vi "NI VeriStand FPGA DMA IO.vi"() -> ()   [LabVIEW 2019]
uses:
  <vilib>/Platform/TimedLoop/XDataNode/wakeup.ctl
  <vilib>/Platform/TimedLoop/XDataNode/XDNodeRunTimeDep.lvlib
  <vilib>/Platform/TimedLoop/XDataNode/nitl_modes.ctl
  <vilib>/Platform/TimedLoop/XDataNode/timing_clust.ctl
  <vilib>/Platform/TimedLoop/XDataNode/XDataNode.xnode
  <vilib>/eio/EIONode/EIONode.xnode
  <vilib>/NI VeriStand/FPGA/NI_VS FPGA Support.lvlib
  <vilib>/eio/EIOMethodNode/EIOMethodNode.xnode
  <vilib>/rvi/eio/common/nirviEmuTemplateMethod_errors.vi
panel:
  in  "Generate IRQ":bool
  in  "Clock Pulse":bool
  in  "Clock Ticked":bool
  in  "Use External Timing":bool
  in  "Write to  RTSI":bool
  in  "Loop Rate (usec)":u32
  in  "Start":bool
  in  "_Low Pulse 7":u32
  in  "_High Pulse 7":u32
  in  "_Low Pulse 5":u32
  in  "_High Pulse 5":u32
  in  "_Low Pulse 6":u32
  in  "_High Pulse 6":u32
  in  "_Low Pulse 4":u32
  in  "_High Pulse 4":u32
  in  "_PWM In 7 timeout":u32=40000
  out "_PWM In 7 High Time":u32
  out "_PWM In 7 Low Time":u32
  in  "_PWM In 6 timeout":u32=40000
  out "_PWM In 6 High Time":u32
  out "_PWM In 6 Low Time":u32
  in  "_PWM In 5 timeout":u32=40000
  out "_PWM In 5 High Time":u32
  out "_PWM In 5 Low Time":u32
  in  "_PWM In 4 timeout":u32=40000
  out "_PWM In 4 High Time":u32
  out "_PWM In 4 Low Time":u32
  in  "_PWM In 3 timeout":u32=40000
  out "_PWM In 3 High Time":u32
  out "_PWM In 3 Low Time":u32
  in  "_PWM In 2 timeout":u32=40000
  out "_PWM In 2 High Time":u32
  out "_PWM In 2 Low Time":u32
  in  "_PWM In 1 timeout":u32=40000
  out "_PWM In 1 High Time":u32
  out "_PWM In 1 Low Time":u32
  in  "_PWM In 0 timeout":u32=40000
  out "_PWM In 0 High Time":u32
  out "_PWM In 0 Low Time":u32
  in  "_Low Pulse 3":u32
  in  "_High Pulse 3":u32
  in  "_Low Pulse 1":u32
  in  "_High Pulse 1":u32
  in  "_Low Pulse 2":u32
  in  "_High Pulse 2":u32
  in  "_Low Pulse 0":u32
  in  "_High Pulse 0":u32
  # "PWM"
  # "Configuration"
  # "Internal Controls"
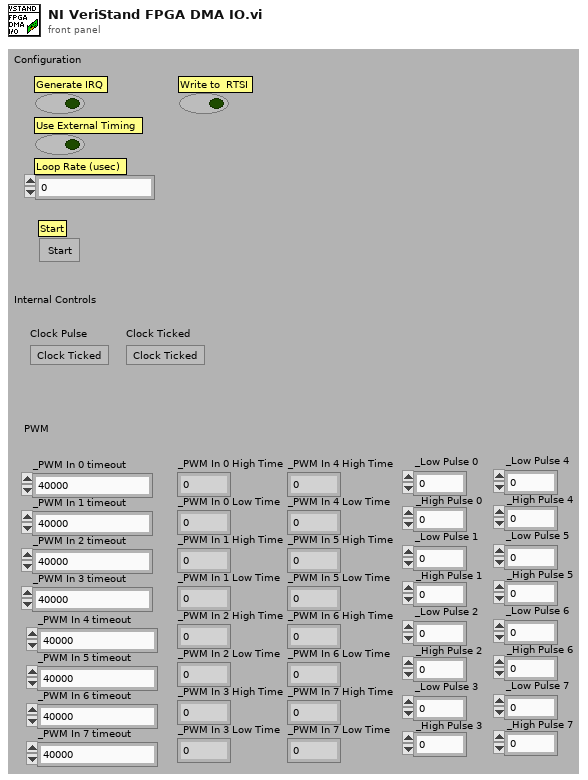
[diagram p1: front panel]
types:
  T1 = typedef "XDNodeRunTimeDep.lvlib/timing_clust.ctl" = cluster{"Expected End [f-1]":u64, "Actual End [f-1]":u64, "Finished Late? [f-1]":bool, "Expected End [i-1]":u64, "Actual End [i-1]":u64, "Finished Late? [i-1]":bool, "Expected Start [i]":u64, "Actual Start [i]":u64, "Expected Start [f]":u64, "Actual Start [f]":u64, "Source Name":string, "Structure Name":string, "Period":i64, "Deadline":i64, "Offset":i64, "Start":i64, "Priority":i32, "Timeout":i32, "Mode":T2, "Wakeup Reason":T3, "Error":errorcluster, "Source Type":string, "Secondary Source Type":string, "Global End Time":u64, "Global Start Time":u64, "Frame Duration":u64, "Iteration Duration":u64, "Assigned CPU":i32, "I/O Scan Engine Mode":u32}
  T2 = typedef "XDNodeRunTimeDep.lvlib/nitl_modes.ctl" = enum32{"No Change", "Process missed periods, maintain original phase", "Discard missed periods, maintain original phase", "Process missed periods, ignore original phase", "Discard missed periods, ignore original phase"}
  T3 = typedef "XDNodeRunTimeDep.lvlib/wakeup.ctl" = enum32{"Normal", "Aborted", "Asynchronous wakeup", "Timing source error", "Timed loop error", "Timeout"}
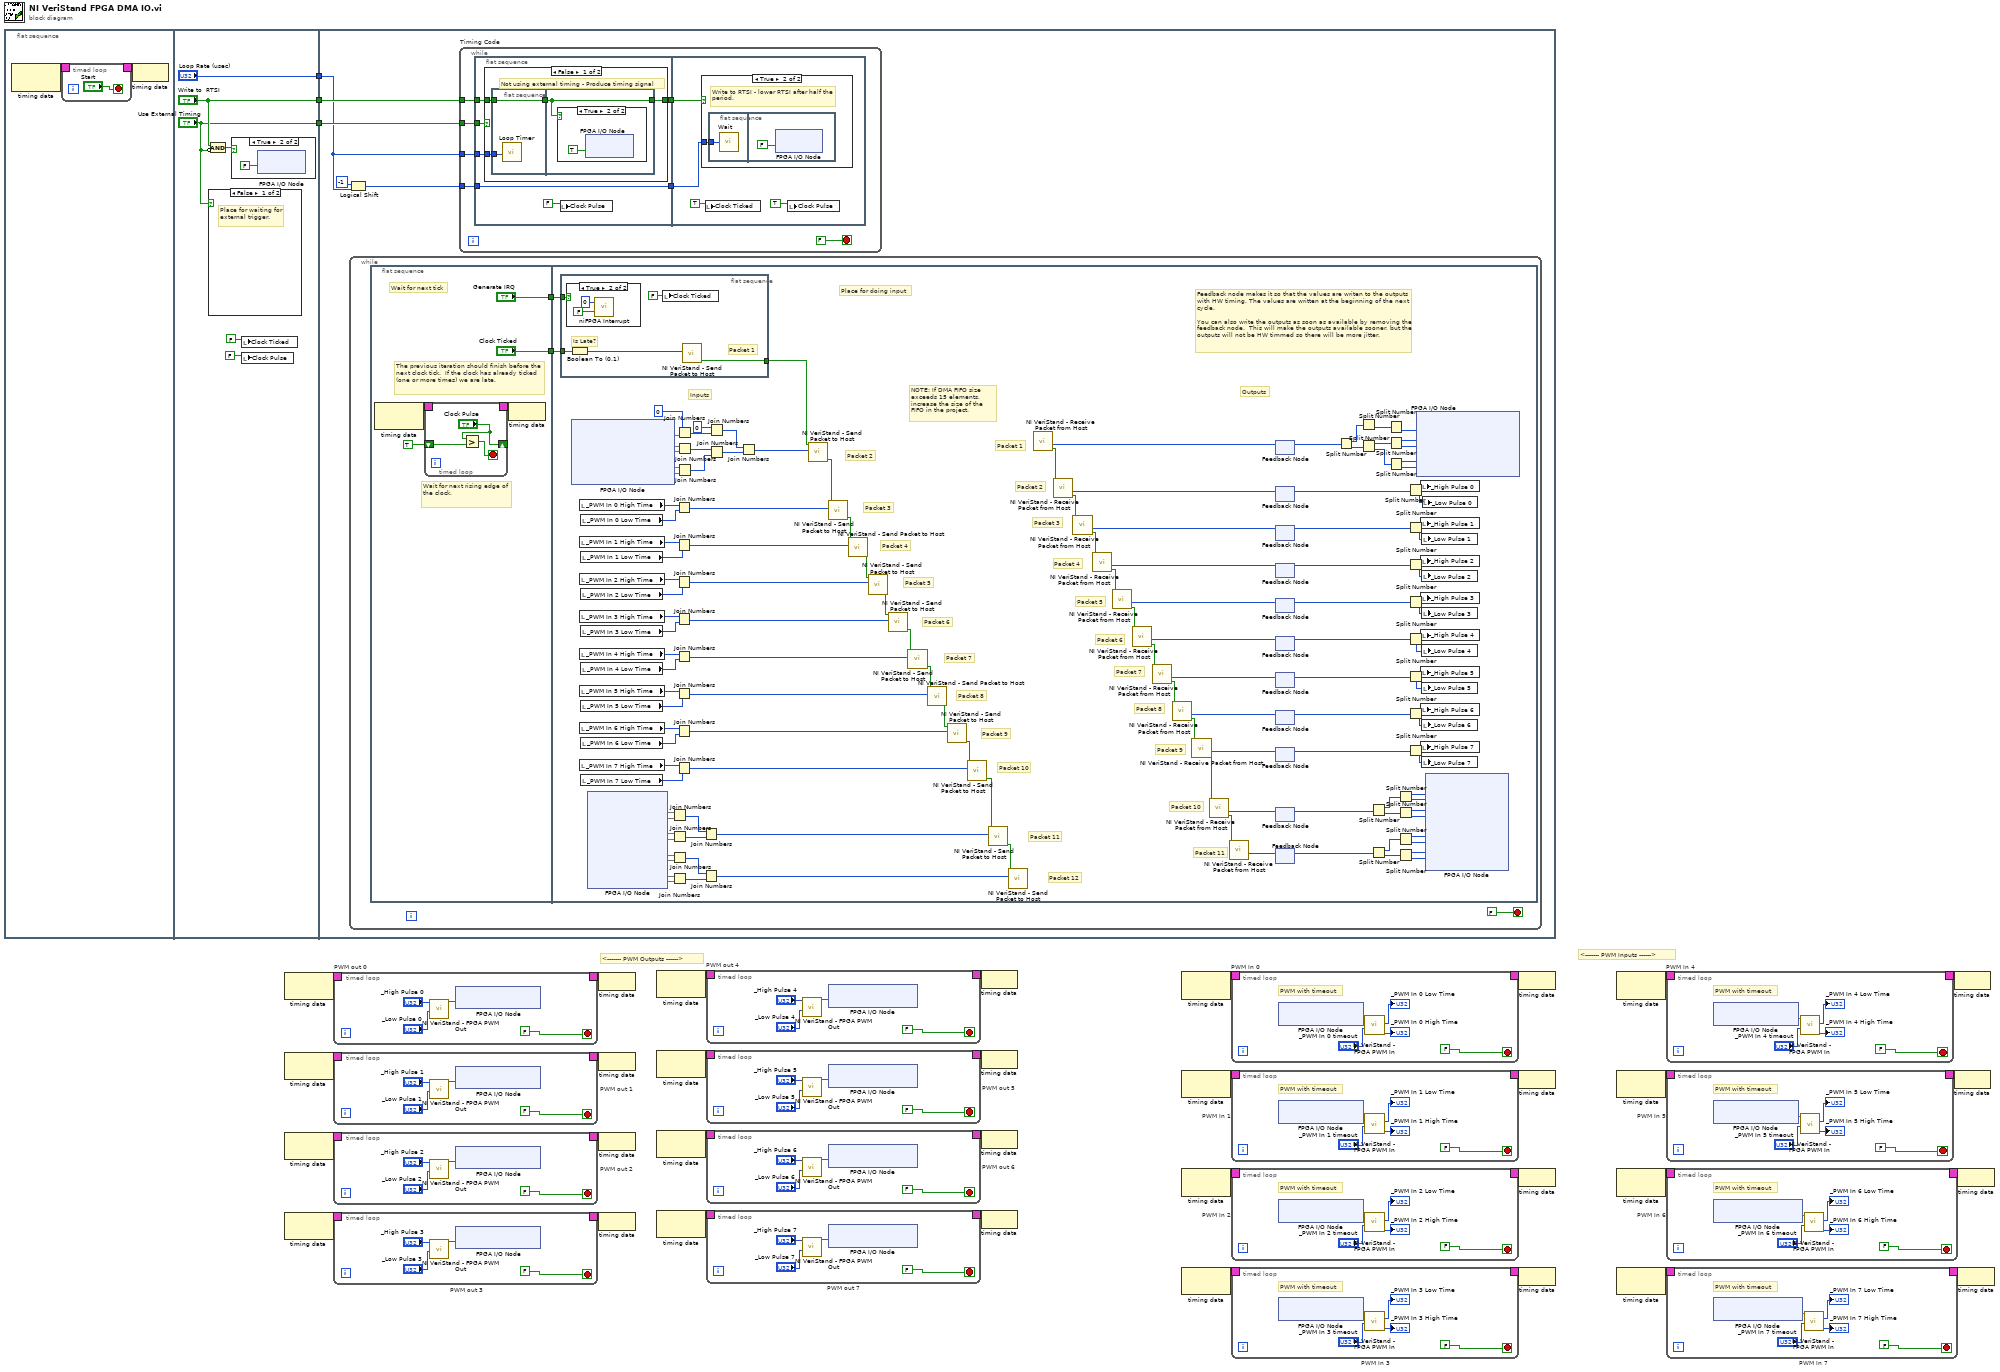
[diagram p0: block diagram]
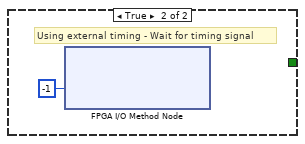
[diagram p5: hidden frame]
diagram:
  # "<------- PWM Outputs ------>"
  # "<------- PWM Inputs ------>"
  n1 = flat-sequence {
    tunnel: ["Use External Timing"] -> w3
    tunnel: ["Write to  RTSI"] -> w2
    tunnel: ["Loop Rate (usec)"] -> w1
    tunnel: w3 -> [w52]
    tunnel: w2 -> [w51]
    tunnel: w1 -> [w50]
    frame #0 {
      n2 = node-c288() -> (w37:T1)  [unwired: 1 out]
      n3 = timed-loop {
        timing: w37 -> [_]
        timing-out: [_] -> w36
        stop <- "Start" stop-if-true
      }
      n4 = node-c288(w36) -> ()
    }
    frame #1 {
      n5 = case shown="False" "Use External Timing" {
        frame False {
          # "Place for waiting for external trigger."
        }
        frame True {
          # "Do not wait on trigger when externally timed."
        }
      }
      n6 = Compound Arithmetic op=AND("Write to  RTSI", invert "Use External Timing") -> (w47:bool)
      n7 = case shown="True" w47 {
        frame False {
        }
        frame True {
          n8 = xnode "FPGA I/O Node"("TRIG0"=FALSE) -> ()  [unwired: 1 in, 1 out]
        }
      }
      n9 = local write "Clock Ticked"(FALSE ("Clock Ticked")) -> ()
      n10 = local write "Clock Pulse"(FALSE ("Clock Ticked")) -> ()
    }
    frame #2 {
      n11 = Logical Shift(y=i8 -1, x=w50) -> (x << y=w53:u32)
      n12 = while {
        stop <- FALSE stop-if-true
        n13 = flat-sequence {
          tunnel: ["Generate IRQ"] -> w85
          tunnel: ["Clock Ticked"] -> w84
          tunnel: w85 -> [w232]
          tunnel: w84 -> [w231]
          frame #0 {
            # "The previous iteration should finish before the next clock tick.  If the clock has already ticked (one or more times) we are late."
            # "Wait for next rising edge of the clock."
            # "Wait for next tick"
            n14 = node-c288() -> (w90:T1)  [unwired: 1 out]
            n15 = timed-loop {
              timing: w90 -> [_]
              timing-out: [_] -> w89
              shift-right: ["Clock Pulse"] -> _
              shift-left: TRUE ("Clock Ticked") -> [w94]
              stop <- w93 stop-if-true
              n16 = Greater?(x="Clock Pulse", y=w94) -> (0:w93:bool)
            }
            n17 = node-c288(w89) -> ()
          }
          frame #1 {
            # "Inputs"
            # "Outputs"
            # "Packet 10"
            # "Packet 9"
            # "Packet 8"
            # "Packet 7"
            # "Packet 6"
            # "Packet 5"
            # "Packet 4"
            # "Packet 3"
            # "Packet 2"
            # "Packet 12"
            # "Packet 11"
            # "Packet 10"
            # "Packet 9"
            # "Packet 8"
            # "Packet 7"
            # "Packet 6"
            # "Packet 5"
            # "Packet 4"
            # "Packet 3"
            # "Packet 2"
            # "Packet 1"
            # "Packet 11"
            # "NOTE: If DMA FIFO size exceeds 15 elements, increase the size of the FIFO in the project."
            # "Feedback node makes it so that the values are writen to the outputs with HW timing. The values are written at the beginning of the next cycle.  \n\nYou can also write the outputs as soon as available by removing the feedback node.  This will make the outputs available sooner, but the outputs will not be HW timmed so there will be more jitter."
            # "Place for doing input"
            n18 = flat-sequence {
              tunnel: w232 -> [w237]
              tunnel: [w235] -> w99
              tunnel: w231 -> [w233]
              frame #0 {
                # "Packet 1"
                # "Is Late?"
                n19 = case shown="True" w237 {
                  frame False {
                  }
                  frame True {
                    n20 = call <vilib>:"niFPGA Interrupt.vi"("Wait Until Cleared (F)"=FALSE ("Wait Until Cleared"), "IRQ Number (0)"=u8 0 ("IRQ Number")) -> ()  [unwired: 1 in]
                  }
                }
                n21 = Boolean To (0,1)(Boolean=w233) -> (0, 1=w236:i16)
                n22 = local write "Clock Ticked"(FALSE ("Clock Ticked")) -> ()
                n23 = call <vilib>:"NI VeriStand - Send Packet to Host.vi"("Element"=w236) -> ("Next"=w235:bool)  [unwired: 1 in, 9 out]
              }
            }
            n24 = xnode "FPGA I/O Node"() -> ("Connector1/DIOPORT4"=w222, "Connector1/DIOPORT3"=w221, "Connector1/DIOPORT2"=w220, "Connector1/DIOPORT1"=w219, "Connector1/DIOPORT0"=w218)  [unwired: 5 in, 5 out]
            n25 = local read "_PWM In 0 High Time"() -> (w208:u32)
            n26 = local read "_PWM In 1 High Time"() -> (w206:u32)
            n27 = local read "_PWM In 2 High Time"() -> (w204:u32)
            n28 = local read "_PWM In 3 High Time"() -> (w202:u32)
            n29 = local read "_PWM In 4 High Time"() -> (w200:u32)
            n30 = local read "_PWM In 5 High Time"() -> (w198:u32)
            n31 = local read "_PWM In 6 High Time"() -> (w196:u32)
            n32 = local read "_PWM In 7 High Time"() -> (w194:u32)
            n33 = local read "_PWM In 0 Low Time"() -> (w207:u32)
            n34 = local read "_PWM In 1 Low Time"() -> (w205:u32)
            n35 = local read "_PWM In 2 Low Time"() -> (w203:u32)
            n36 = local read "_PWM In 3 Low Time"() -> (w201:u32)
            n37 = local read "_PWM In 4 Low Time"() -> (w199:u32)
            n38 = local read "_PWM In 5 Low Time"() -> (w197:u32)
            n39 = local read "_PWM In 6 Low Time"() -> (w195:u32)
            n40 = local read "_PWM In 7 Low Time"() -> (w193:u32)
            n41 = xnode "FPGA I/O Node"() -> ("Connector0/AI3"=w230, "Connector0/AI2"=w229, "Connector0/AI1"=w228, "Connector0/AI0"=w227, "Connector0/AI7"=w226, "Connector0/AI6"=w225, "Connector0/AI5"=w224, "Connector0/AI4"=w223)  [unwired: 8 in, 8 out]
            n42 = Join Numbers(hi=w230, lo=w229) -> ((hi.lo)=w213:u32)
            n43 = Join Numbers(hi=w228, lo=w227) -> ((hi.lo)=w214:u32)
            n44 = Join Numbers(hi=w226, lo=w225) -> ((hi.lo)=w211:u32)
            n45 = Join Numbers(hi=w224, lo=w223) -> ((hi.lo)=w212:u32)
            n46 = Join Numbers(hi=w208, lo=w207) -> ((hi.lo)=w149:u64)
            n47 = Join Numbers(hi=w206, lo=w205) -> ((hi.lo)=w148:u64)
            n48 = Join Numbers(hi=w204, lo=w203) -> ((hi.lo)=w147:u64)
            n49 = Join Numbers(hi=w202, lo=w201) -> ((hi.lo)=w146:u64)
            n50 = Join Numbers(hi=w200, lo=w199) -> ((hi.lo)=w145:u64)
            n51 = Join Numbers(hi=w198, lo=w197) -> ((hi.lo)=w144:u64)
            n52 = Join Numbers(hi=w196, lo=w195) -> ((hi.lo)=w143:u64)
            n53 = Join Numbers(hi=w194, lo=w193) -> ((hi.lo)=w142:u64)
            n54 = Join Numbers(hi=u8 0, lo=w222) -> ((hi.lo)=w217:u16)
            n55 = Join Numbers(hi=w221, lo=w220) -> ((hi.lo)=w216:u32)
            n56 = Join Numbers(hi=w219, lo=w218) -> ((hi.lo)=w215:u32)
            n57 = Join Numbers(hi=w213, lo=w214) -> ((hi.lo)=w152:u64)
            n58 = Join Numbers(hi=w211, lo=w212) -> ((hi.lo)=w151:u64)
            n59 = Join Numbers(hi=u16 0, lo=w217) -> ((hi.lo)=w210:u32)
            n60 = Join Numbers(hi=w216, lo=w215) -> ((hi.lo)=w209:u64)
            n61 = Join Numbers(hi=w210, lo=w209) -> ((hi.lo)=w150:u64)
            n62 = call <vilib>:"NI VeriStand - Send Packet to Host.vi"("Element"=w150, "Prev"=w99) -> ("Next"=w109:bool)  [unwired: 1 in, 8 out]
            n63 = call <vilib>:"NI VeriStand - Send Packet to Host.vi"("Element"=w149, "Prev"=w109) -> ("Next"=w108:bool)  [unwired: 1 in, 8 out]
            n64 = call <vilib>:"NI VeriStand - Send Packet to Host.vi"("Element"=w148, "Prev"=w108) -> ("Next"=w107:bool)  [unwired: 1 in, 8 out]
            n65 = call <vilib>:"NI VeriStand - Send Packet to Host.vi"("Element"=w147, "Prev"=w107) -> ("Next"=w106:bool)  [unwired: 1 in, 8 out]
            n66 = call <vilib>:"NI VeriStand - Send Packet to Host.vi"("Element"=w146, "Prev"=w106) -> ("Next"=w105:bool)  [unwired: 1 in, 8 out]
            n67 = call <vilib>:"NI VeriStand - Send Packet to Host.vi"("Element"=w145, "Prev"=w105) -> ("Next"=w104:bool)  [unwired: 1 in, 8 out]
            n68 = call <vilib>:"NI VeriStand - Send Packet to Host.vi"("Element"=w144, "Prev"=w104) -> ("Next"=w103:bool)  [unwired: 1 in, 8 out]
            n69 = call <vilib>:"NI VeriStand - Send Packet to Host.vi"("Element"=w143, "Prev"=w103) -> ("Next"=w102:bool)  [unwired: 1 in, 8 out]
            n70 = call <vilib>:"NI VeriStand - Send Packet to Host.vi"("Element"=w142, "Prev"=w102) -> ("Next"=w101:bool)  [unwired: 1 in, 8 out]
            n71 = call <vilib>:"NI VeriStand - Send Packet to Host.vi"("Element"=w152, "Prev"=w101) -> ("Next"=w110:bool)  [unwired: 1 in, 8 out]
            n72 = call <vilib>:"NI VeriStand - Send Packet to Host.vi"("Element"=w151, "Prev"=w110) -> ()  [unwired: 1 in, 9 out]
            n73 = call <vilib>:"NI VeriStand - Receive Packet from Host.vi"() -> ("Next"=w118:bool, "Element"=w139:u64)  [unwired: 2 in, 8 out]
            n74 = call <vilib>:"NI VeriStand - Receive Packet from Host.vi"("Prev"=w118) -> ("Next"=w117:bool, "Element"=w138:u64)  [unwired: 1 in, 8 out]
            n75 = call <vilib>:"NI VeriStand - Receive Packet from Host.vi"("Prev"=w117) -> ("Next"=w116:bool, "Element"=w137:u64)  [unwired: 1 in, 8 out]
            n76 = call <vilib>:"NI VeriStand - Receive Packet from Host.vi"("Prev"=w116) -> ("Next"=w115:bool, "Element"=w135:u64)  [unwired: 1 in, 8 out]
            n77 = call <vilib>:"NI VeriStand - Receive Packet from Host.vi"("Prev"=w115) -> ("Next"=w114:bool, "Element"=w134:u64)  [unwired: 1 in, 8 out]
            n78 = call <vilib>:"NI VeriStand - Receive Packet from Host.vi"("Prev"=w114) -> ("Next"=w113:bool, "Element"=w133:u64)  [unwired: 1 in, 8 out]
            n79 = call <vilib>:"NI VeriStand - Receive Packet from Host.vi"("Prev"=w113) -> ("Next"=w112:bool, "Element"=w132:u64)  [unwired: 1 in, 8 out]
            n80 = call <vilib>:"NI VeriStand - Receive Packet from Host.vi"("Prev"=w112) -> ("Next"=w111:bool, "Element"=w131:u64)  [unwired: 1 in, 8 out]
            n81 = call <vilib>:"NI VeriStand - Receive Packet from Host.vi"("Prev"=w111) -> ("Next"=w100:bool, "Element"=w136:u64)  [unwired: 1 in, 8 out]
            n82 = call <vilib>:"NI VeriStand - Receive Packet from Host.vi"("Prev"=w100) -> ("Next"=w119:bool, "Element"=w141:u64)  [unwired: 9 out]
            n83 = call <vilib>:"NI VeriStand - Receive Packet from Host.vi"("Prev"=w119) -> ("Element"=w140:u64)  [unwired: 1 in, 9 out]
            n84 = feedback-in #1(w139) -> ()
            n85 = feedback #1() -> (w128:u64)  [unwired: 1 out]
            n86 = feedback-in #2(w138) -> ()
            n87 = feedback #2() -> (w127:u64)  [unwired: 1 out]
            n88 = feedback-in #3(w137) -> ()
            n89 = feedback #3() -> (w126:u64)  [unwired: 1 out]
            n90 = feedback-in #4(w135) -> ()
            n91 = feedback #4() -> (w125:u64)  [unwired: 1 out]
            n92 = feedback-in #5(w134) -> ()
            n93 = feedback #5() -> (w124:u64)  [unwired: 1 out]
            n94 = feedback-in #6(w133) -> ()
            n95 = feedback #6() -> (w123:u64)  [unwired: 1 out]
            n96 = feedback-in #7(w132) -> ()
            n97 = feedback #7() -> (w122:u64)  [unwired: 1 out]
            n98 = feedback-in #8(w131) -> ()
            n99 = feedback #8() -> (w121:u64)  [unwired: 1 out]
            n100 = feedback-in #9(w136) -> ()
            n101 = feedback #9() -> (w120:u64)  [unwired: 1 out]
            n102 = feedback-in #10(w141) -> ()
            n103 = feedback #10() -> (w130:u64)  [unwired: 1 out]
            n104 = feedback-in #11(w140) -> ()
            n105 = feedback #11() -> (w129:u64)  [unwired: 1 out]
            n106 = Split Number(x=w128) -> (hi(x)=w175:u32, lo(x)=w174:u32)
            n107 = Split Number(x=w175) -> (lo(x)=w180:u16)  [unwired: 1 out]
            n108 = Split Number(x=w174) -> (hi(x)=w182:u16, lo(x)=w181:u16)
            n109 = Split Number(x=w130) -> (hi(x)=w178:u32, lo(x)=w179:u32)
            n110 = Split Number(x=w129) -> (hi(x)=w177:u32, lo(x)=w176:u32)
            n111 = Split Number(x=w180) -> (lo(x)=w153:u8)  [unwired: 1 out]
            n112 = Split Number(x=w182) -> (hi(x)=w154:u8, lo(x)=w155:u8)
            n113 = Split Number(x=w181) -> (hi(x)=w156:u8, lo(x)=w157:u8)
            n114 = Split Number(x=w178) -> (hi(x)=w183:u16, lo(x)=w190:u16)
            n115 = Split Number(x=w179) -> (hi(x)=w189:u16, lo(x)=w188:u16)
            n116 = Split Number(x=w177) -> (hi(x)=w187:u16, lo(x)=w186:u16)
            n117 = Split Number(x=w176) -> (hi(x)=w185:u16, lo(x)=w184:u16)
            n118 = Split Number(x=w127) -> (hi(x)=w173:u32, lo(x)=w172:u32)
            n119 = Split Number(x=w126) -> (hi(x)=w171:u32, lo(x)=w170:u32)
            n120 = Split Number(x=w125) -> (hi(x)=w169:u32, lo(x)=w168:u32)
            n121 = Split Number(x=w124) -> (hi(x)=w167:u32, lo(x)=w166:u32)
            n122 = Split Number(x=w123) -> (hi(x)=w165:u32, lo(x)=w164:u32)
            n123 = Split Number(x=w122) -> (hi(x)=w163:u32, lo(x)=w162:u32)
            n124 = Split Number(x=w121) -> (hi(x)=w161:u32, lo(x)=w160:u32)
            n125 = Split Number(x=w120) -> (hi(x)=w159:u32, lo(x)=w158:u32)
            n126 = xnode "FPGA I/O Node"("Connector2/DIOPORT4"=w153, "Connector2/DIOPORT3"=w154, "Connector2/DIOPORT2"=w155, "Connector2/DIOPORT1"=w156, "Connector2/DIOPORT0"=w157) -> ()  [unwired: 5 in, 5 out]
            n127 = local write "_High Pulse 0"(w173) -> ()
            n128 = local write "_High Pulse 1"(w171) -> ()
            n129 = local write "_High Pulse 2"(w169) -> ()
            n130 = local write "_High Pulse 3"(w167) -> ()
            n131 = local write "_High Pulse 4"(w165) -> ()
            n132 = local write "_High Pulse 5"(w163) -> ()
            n133 = local write "_High Pulse 6"(w161) -> ()
            n134 = local write "_High Pulse 7"(w159) -> ()
            n135 = local write "_Low Pulse 1"(w170) -> ()
            n136 = local write "_Low Pulse 2"(w168) -> ()
            n137 = local write "_Low Pulse 3"(w166) -> ()
            n138 = local write "_Low Pulse 4"(w164) -> ()
            n139 = local write "_Low Pulse 5"(w162) -> ()
            n140 = local write "_Low Pulse 6"(w160) -> ()
            n141 = local write "_Low Pulse 7"(w158) -> ()
            n142 = local write "_Low Pulse 0"(w172) -> ()
            n143 = xnode "FPGA I/O Node"("Connector0/AO3"=w183, "Connector0/AO2"=w190, "Connector0/AO1"=w189, "Connector0/AO0"=w188, "Connector0/AO7"=w187, "Connector0/AO6"=w186, "Connector0/AO5"=w185, "Connector0/AO4"=w184) -> ()  [unwired: 8 in, 8 out]
          }
        }
      }
      n144 = while "Timing Code" {
        tunnel: w53 -> [w61]
        tunnel: w50 -> [w60]
        tunnel: w52 -> [w59]
        tunnel: w51 -> [w58]
        stop <- FALSE stop-if-true
        n145 = flat-sequence {
          tunnel: w61 -> [w64]
          tunnel: w60 -> [w67]
          tunnel: w59 -> [w66]
          tunnel: w58 -> [w65]
          tunnel: [w64] -> w56
          tunnel: [w62] -> w55
          tunnel: w56 -> [w80]
          tunnel: w55 -> [w77]
          frame #0 {
            n146 = case shown="False" w66 {
              tunnel: w67 -> [w71 _]
              tunnel: w65 -> [w69 _]
              tunnel: [w68 _] -> w62
              frame False {
                # "Not using external timing - Produce timing signal"
                n147 = flat-sequence {
                  tunnel: [w72] -> w70
                  tunnel: w71 -> [w73]
                  tunnel: w69 -> [w72]
                  tunnel: w70 -> [w74]
                  tunnel: [w74] -> w68
                  frame #0 {
                    n148 = call "Loop Timer"("Count(uSec)"=w73) -> ()  [unwired: 1 out]
                  }
                  frame #1 {
                    n149 = case shown="True" w74 {
                      frame False {
                      }
                      frame True {
                        n150 = xnode "FPGA I/O Node"("TRIG0"=TRUE) -> ()  [unwired: 1 in, 1 out]
                      }
                    }
                  }
                }
              }
              frame True {
                # "Using external timing - Wait for timing signal"
                n151 = xnode "FPGA I/O Method Node"("Timeout"=-1) -> ()  [unwired: 1 in, 2 out]
              }
            }
            n152 = local write "Clock Pulse"(FALSE ("Clock Ticked")) -> ()
          }
          frame #1 {
            n153 = case shown="True" w77 {
              tunnel: w80 -> [_ w81]
              frame False {
              }
              frame True {
                # "Write to RTSI - lower RTSI after half the period."
                n154 = flat-sequence {
                  tunnel: w81 -> [w82]
                  frame #0 {
                    n155 = call "Wait"("Count(uSec)"=w82) -> ()  [unwired: 1 out]
                  }
                  frame #1 {
                    n156 = xnode "FPGA I/O Node"("TRIG0"=FALSE) -> ()  [unwired: 1 in, 1 out]
                  }
                }
              }
            }
            n157 = local write "Clock Ticked"(TRUE ("Clock Ticked")) -> ()
            n158 = local write "Clock Pulse"(TRUE ("Clock Ticked")) -> ()
          }
        }
      }
    }
  }
  n159 = node-c288() -> (w35:T1)  [unwired: 1 out]
  n160 = node-c288() -> (w31:T1)  [unwired: 1 out]
  n161 = node-c288() -> (w33:T1)  [unwired: 1 out]
  n162 = node-c288() -> (w29:T1)  [unwired: 1 out]
  n163 = timed-loop "PWM out 0" {
    timing: w35 -> [_]
    timing-out: [_] -> w34
    stop <- FALSE stop-if-true
    n164 = call <vilib>:"NI VeriStand - FPGA PWM Out.vi"("_Low Time"="_Low Pulse 0", "_High Time"="_High Pulse 0") -> ("Output"=w242:bool)  [unwired: 1 in, 8 out]
    n165 = xnode "FPGA I/O Node"("Connector0/DIO4"=w242) -> ()  [unwired: 1 in, 1 out]
  }
  n166 = timed-loop "PWM out 1" {
    timing: w31 -> [_]
    timing-out: [_] -> w30
    stop <- FALSE stop-if-true
    n167 = call <vilib>:"NI VeriStand - FPGA PWM Out.vi"("_Low Time"="_Low Pulse 1", "_High Time"="_High Pulse 1") -> ("Output"=w246:bool)  [unwired: 1 in, 8 out]
    n168 = xnode "FPGA I/O Node"("Connector0/DIO5"=w246) -> ()  [unwired: 1 in, 1 out]
  }
  n169 = timed-loop "PWM out 2" {
    timing: w33 -> [_]
    timing-out: [_] -> w32
    stop <- FALSE stop-if-true
    n170 = call <vilib>:"NI VeriStand - FPGA PWM Out.vi"("_Low Time"="_Low Pulse 2", "_High Time"="_High Pulse 2") -> ("Output"=w254:bool)  [unwired: 1 in, 8 out]
    n171 = xnode "FPGA I/O Node"("Connector0/DIO6"=w254) -> ()  [unwired: 1 in, 1 out]
  }
  n172 = timed-loop "PWM out 3" {
    timing: w29 -> [_]
    timing-out: [_] -> w28
    stop <- FALSE stop-if-true
    n173 = call <vilib>:"NI VeriStand - FPGA PWM Out.vi"("_Low Time"="_Low Pulse 3", "_High Time"="_High Pulse 3") -> ("Output"=w261:bool)  [unwired: 1 in, 8 out]
    n174 = xnode "FPGA I/O Node"("Connector0/DIO7"=w261) -> ()  [unwired: 1 in, 1 out]
  }
  n175 = node-c288(w34) -> ()
  n176 = node-c288(w30) -> ()
  n177 = node-c288(w32) -> ()
  n178 = node-c288(w28) -> ()
  n179 = node-c288() -> (w11:T1)  [unwired: 1 out]
  n180 = node-c288() -> (w7:T1)  [unwired: 1 out]
  n181 = node-c288() -> (w9:T1)  [unwired: 1 out]
  n182 = node-c288() -> (w5:T1)  [unwired: 1 out]
  n183 = timed-loop "PWM out 4" {
    timing: w11 -> [_]
    timing-out: [_] -> w10
    stop <- FALSE stop-if-true
    n184 = call <vilib>:"NI VeriStand - FPGA PWM Out.vi"("_Low Time"="_Low Pulse 4", "_High Time"="_High Pulse 4") -> ("Output"=w266:bool)  [unwired: 1 in, 8 out]
    n185 = xnode "FPGA I/O Node"("Connector0/DIO12"=w266) -> ()  [unwired: 1 in, 1 out]
  }
  n186 = timed-loop "PWM out 5" {
    timing: w7 -> [_]
    timing-out: [_] -> w6
    stop <- FALSE stop-if-true
    n187 = call <vilib>:"NI VeriStand - FPGA PWM Out.vi"("_Low Time"="_Low Pulse 5", "_High Time"="_High Pulse 5") -> ("Output"=w270:bool)  [unwired: 1 in, 8 out]
    n188 = xnode "FPGA I/O Node"("Connector0/DIO13"=w270) -> ()  [unwired: 1 in, 1 out]
  }
  n189 = timed-loop "PWM out 6" {
    timing: w9 -> [_]
    timing-out: [_] -> w8
    stop <- FALSE stop-if-true
    n190 = call <vilib>:"NI VeriStand - FPGA PWM Out.vi"("_Low Time"="_Low Pulse 6", "_High Time"="_High Pulse 6") -> ("Output"=w278:bool)  [unwired: 1 in, 8 out]
    n191 = xnode "FPGA I/O Node"("Connector0/DIO14"=w278) -> ()  [unwired: 1 in, 1 out]
  }
  n192 = timed-loop "PWM out 7" {
    timing: w5 -> [_]
    timing-out: [_] -> w4
    stop <- FALSE stop-if-true
    n193 = call <vilib>:"NI VeriStand - FPGA PWM Out.vi"("_Low Time"="_Low Pulse 7", "_High Time"="_High Pulse 7") -> ("Output"=w282:bool)  [unwired: 1 in, 8 out]
    n194 = xnode "FPGA I/O Node"("Connector0/DIO15"=w282) -> ()  [unwired: 1 in, 1 out]
  }
  n195 = node-c288(w10) -> ()
  n196 = node-c288(w6) -> ()
  n197 = node-c288(w8) -> ()
  n198 = node-c288(w4) -> ()
  n199 = node-c288() -> (w27:T1)  [unwired: 1 out]
  n200 = node-c288() -> (w25:T1)  [unwired: 1 out]
  n201 = node-c288() -> (w23:T1)  [unwired: 1 out]
  n202 = node-c288() -> (w21:T1)  [unwired: 1 out]
  n203 = timed-loop "PWM In 0" {
    timing: w27 -> [_]
    timing-out: [_] -> w26
    stop <- FALSE stop-if-true
    # "PWM with timeout"
    n204 = xnode "FPGA I/O Node"() -> ("Connector0/DIO0"=w291)  [unwired: 1 in, 1 out]
    n205 = call <vilib>:"NI VeriStand - FPGA PWM In.vi"("Time Out"="_PWM In 0 timeout", "Value"=w291) -> ("High time"=→"_PWM In 0 High Time":u32, "Low Time"=→"_PWM In 0 Low Time":u32)  [unwired: 8 out]
  }
  n206 = timed-loop "PWM In 1" {
    timing: w25 -> [_]
    timing-out: [_] -> w24
    stop <- FALSE stop-if-true
    # "PWM with timeout"
    n207 = xnode "FPGA I/O Node"() -> ("Connector0/DIO1"=w298)  [unwired: 1 in, 1 out]
    n208 = call <vilib>:"NI VeriStand - FPGA PWM In.vi"("Time Out"="_PWM In 1 timeout", "Value"=w298) -> ("High time"=→"_PWM In 1 High Time":u32, "Low Time"=→"_PWM In 1 Low Time":u32)  [unwired: 8 out]
  }
  n209 = timed-loop "PWM In 2" {
    timing: w23 -> [_]
    timing-out: [_] -> w22
    stop <- FALSE stop-if-true
    # "PWM with timeout"
    n210 = xnode "FPGA I/O Node"() -> ("Connector0/DIO2"=w305)  [unwired: 1 in, 1 out]
    n211 = call <vilib>:"NI VeriStand - FPGA PWM In.vi"("Time Out"="_PWM In 2 timeout", "Value"=w305) -> ("High time"=→"_PWM In 2 High Time":u32, "Low Time"=→"_PWM In 2 Low Time":u32)  [unwired: 8 out]
  }
  n212 = timed-loop "PWM In 3" {
    timing: w21 -> [_]
    timing-out: [_] -> w20
    stop <- FALSE stop-if-true
    # "PWM with timeout"
    n213 = xnode "FPGA I/O Node"() -> ("Connector0/DIO3"=w312)  [unwired: 1 in, 1 out]
    n214 = call <vilib>:"NI VeriStand - FPGA PWM In.vi"("Time Out"="_PWM In 3 timeout", "Value"=w312) -> ("High time"=→"_PWM In 3 High Time":u32, "Low Time"=→"_PWM In 3 Low Time":u32)  [unwired: 8 out]
  }
  n215 = node-c288(w26) -> ()
  n216 = node-c288(w24) -> ()
  n217 = node-c288(w22) -> ()
  n218 = node-c288(w20) -> ()
  n219 = node-c288() -> (w19:T1)  [unwired: 1 out]
  n220 = node-c288() -> (w17:T1)  [unwired: 1 out]
  n221 = node-c288() -> (w15:T1)  [unwired: 1 out]
  n222 = node-c288() -> (w13:T1)  [unwired: 1 out]
  n223 = timed-loop "PWM In 4" {
    timing: w19 -> [_]
    timing-out: [_] -> w18
    stop <- FALSE stop-if-true
    # "PWM with timeout"
    n224 = xnode "FPGA I/O Node"() -> ("Connector0/DIO8"=w319)  [unwired: 1 in, 1 out]
    n225 = call <vilib>:"NI VeriStand - FPGA PWM In.vi"("Time Out"="_PWM In 4 timeout", "Value"=w319) -> ("High time"=→"_PWM In 4 High Time":u32, "Low Time"=→"_PWM In 4 Low Time":u32)  [unwired: 8 out]
  }
  n226 = timed-loop "PWM In 5" {
    timing: w17 -> [_]
    timing-out: [_] -> w16
    stop <- FALSE stop-if-true
    # "PWM with timeout"
    n227 = xnode "FPGA I/O Node"() -> ("Connector0/DIO9"=w326)  [unwired: 1 in, 1 out]
    n228 = call <vilib>:"NI VeriStand - FPGA PWM In.vi"("Time Out"="_PWM In 5 timeout", "Value"=w326) -> ("High time"=→"_PWM In 5 High Time":u32, "Low Time"=→"_PWM In 5 Low Time":u32)  [unwired: 8 out]
  }
  n229 = timed-loop "PWM In 6" {
    timing: w15 -> [_]
    timing-out: [_] -> w14
    stop <- FALSE stop-if-true
    # "PWM with timeout"
    n230 = xnode "FPGA I/O Node"() -> ("Connector0/DIO10"=w333)  [unwired: 1 in, 1 out]
    n231 = call <vilib>:"NI VeriStand - FPGA PWM In.vi"("Time Out"="_PWM In 6 timeout", "Value"=w333) -> ("High time"=→"_PWM In 6 High Time":u32, "Low Time"=→"_PWM In 6 Low Time":u32)  [unwired: 8 out]
  }
  n232 = timed-loop "PWM In 7" {
    timing: w13 -> [_]
    timing-out: [_] -> w12
    stop <- FALSE stop-if-true
    # "PWM with timeout"
    n233 = xnode "FPGA I/O Node"() -> ("Connector0/DIO11"=w340)  [unwired: 1 in, 1 out]
    n234 = call <vilib>:"NI VeriStand - FPGA PWM In.vi"("Time Out"="_PWM In 7 timeout", "Value"=w340) -> ("High time"=→"_PWM In 7 High Time":u32, "Low Time"=→"_PWM In 7 Low Time":u32)  [unwired: 8 out]
  }
  n235 = node-c288(w18) -> ()
  n236 = node-c288(w16) -> ()
  n237 = node-c288(w14) -> ()
  n238 = node-c288(w12) -> ()
